vi "TF Status.vi"() -> ()   [LabVIEW 2021]
uses:
  Controls/Tube Feeder.ctl
panel:
  out "TF Status":T1
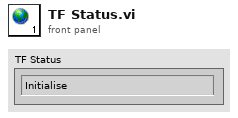
[diagram p1: front panel]
types:
  T1 = typedef "Tube Feeder.ctl" = enum16{"Initialise", "Gate Open", "Wait for Delay", "Gate Close", "Done", "Error"}
diagram:
